vi "shutters activate.vi"() -> ()   [LabVIEW 2011]
doc: "Allows manual operation of laser and camera shutters on h-nu microscope"
uses:
  h-nu-ixon/Laser type.ctt
  h-nu-ixon/Emission filters.ctl
  h-nu-ixon/Filter wheel settings globals.vi
  hardware status globals.vi
panel:
  in  "L0 off1 2":bool
  in  "L0 ON 5":bool
  in  "Emission filter wheel":T1
  out "Status":bool
  in  "C off":bool
  in  "C ON":bool
  out "error out":errorcluster
  in  "All Lasers Off":bool
  in  "L0 off 4":bool
  in  "L0 off 3":bool
  in  "L0 off1":bool
  in  "L0 off 0":bool
  in  "L0 ON 4":bool
  in  "L0 ON 3":bool
  in  "L0 ON 2":bool
  in  "Stop":bool
  in  "L0 ON":bool
  out "Lasers Shutters Status":cluster{"Laser":T2, "Status":bool}[](array[cluster])=[{"Laser"=enum."Blue 488 nm", "Status"=FALSE}, {"Laser"=enum."Green 532 nm", "Status"=FALSE}, {"Laser"=enum."Orange 594 nm", "Status"=FALSE}, {"Laser"=enum."Red 633 nm", "Status"=FALSE}, {"Laser"=enum."IR 780", "Status"=FALSE}]
  # "Open"
  # "Close"
  # "Camera"
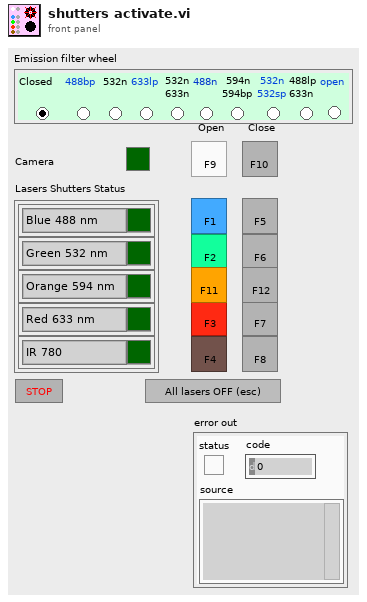
[diagram p1: front panel]
types:
  T1 = typedef "Emission filters.ctl" = enum32{" Closed ", "488bp ", "532n", "633lp ", "532n\n633n", "488n", "594n\n594bp", "532n\n532sp", "488lp\n633n", "open"}
  T2 = typedef "Laser type.ctt" = enum16{"Blue 488 nm", "Green 532 nm", "Orange 594 nm", "Red 633 nm", "IR 780"}
  T3 = enum16{"Blue 488 nm", "Green 532 nm", "Orange 594 nm", "Red 633 nm", "IR 780"}
  T4 = typedef "shutters status.ctl" = cluster{"Laser":T2, "Status":bool}[]
  T5 = enum16{"Blue 488 nm", "Green 532 nm", "Orange 594 nm", "Red 633 nm", "IR 780"}[]
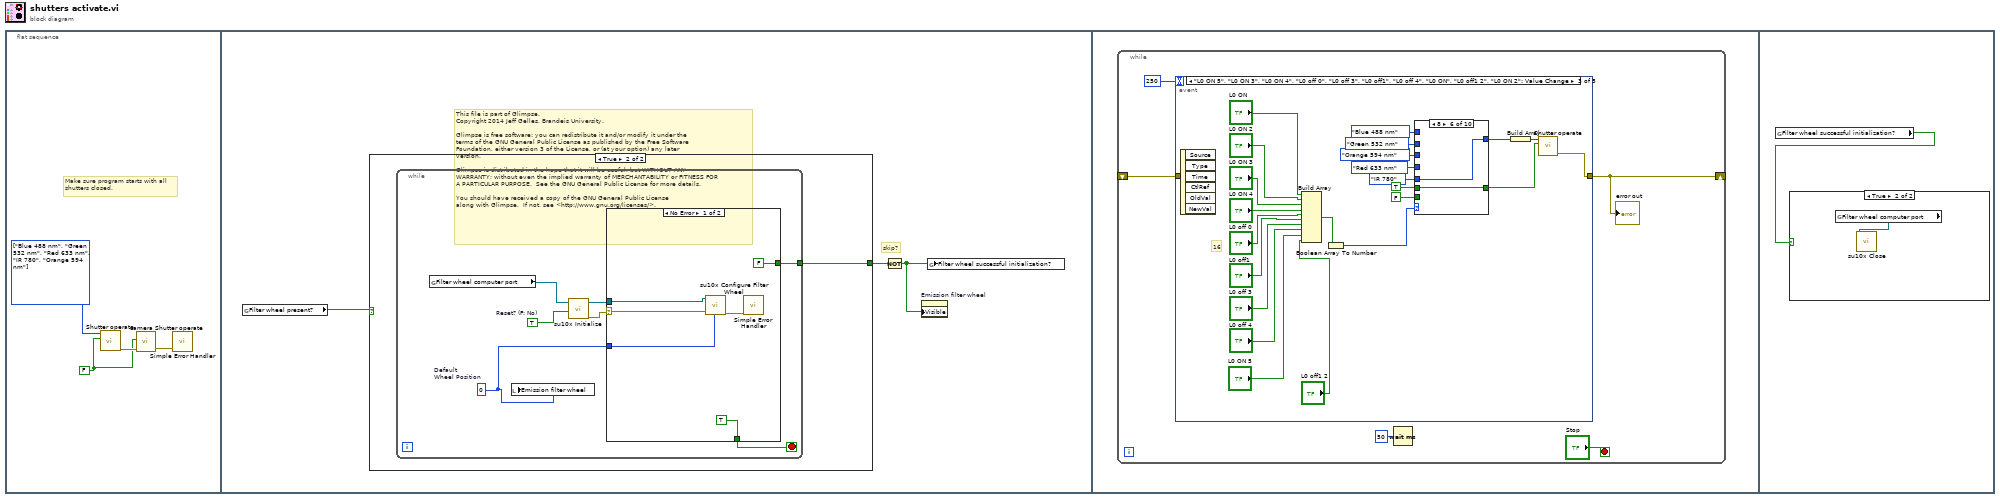
[diagram p0: block diagram]
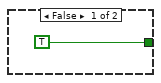
[diagram p2: hidden frame]
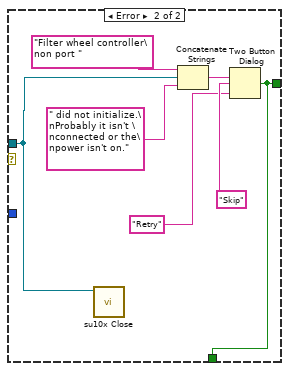
[diagram p3: hidden frame]
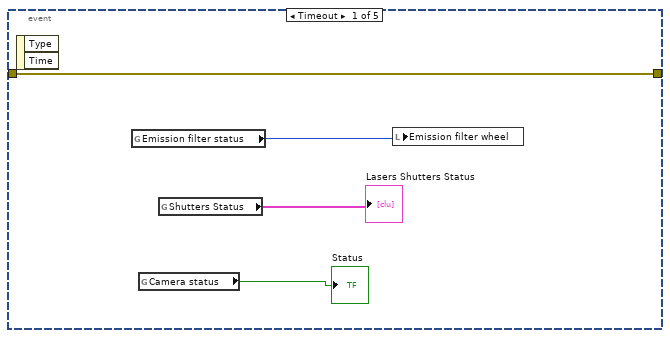
[diagram p4: hidden frame]
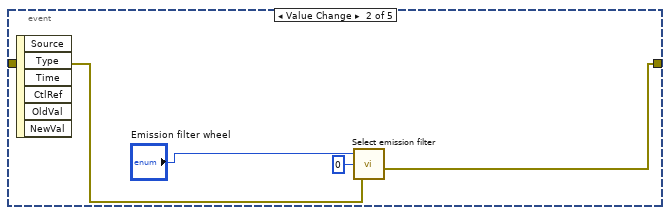
[diagram p5: hidden frame]
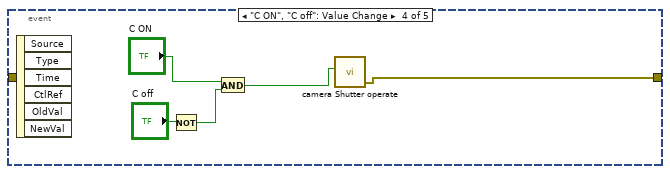
[diagram p15: hidden frame]
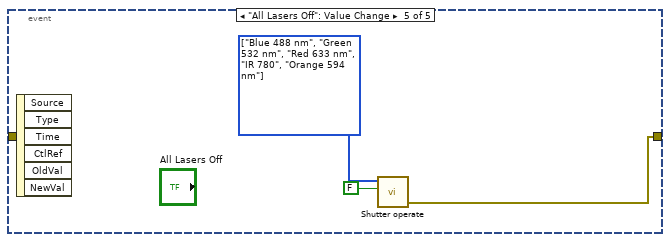
[diagram p16: hidden frame]
diagram:
  # "This file is part of Glimpse. \nCopyright 2014 Jeff Gelles, Brandeis University.    \n\nGlimpse is free software: you can redistribute it and/or modify it under the \nterms of the GNU General Public License as published by the Free Software \nFoundation, either version 3 of the License, or (at your option) any later \nversion.\n\nGlimpse is distributed in the hope that it will be useful, but WITHOUT ANY \nWARRANTY; without even the implied warranty of MERCHANTABILITY or FITNESS FOR \nA PARTICULAR PURPOSE.  See the GNU General Public License for more details.\n\nYou should have received a copy of the GNU General Public License\nalong with Glimpse.  If not, see <http://www.gnu.org/licenses/>."
  n1 = flat-sequence {
    frame #0 {
      w4 = T2[] [enum."Blue 488 nm", enum."Green 532 nm", enum."Red 633 nm", enum."IR 780", enum."Orange 594 nm"] items=["Blue 488 nm", "Green 532 nm", "Orange 594 nm", "Red 633 nm", "IR 780"] ("Shutters")
      w1 = FALSE
      # "Make sure program starts with all\nshutters closed."
      n2 = call "Shutter operate.vi"("Shutters"=w4, 2:w1) -> ("error out"=w3:errorcluster)  [unwired: 1 in, 5 out]
      n3 = call "camera Shutter operate.vi"("Open?"=w1, "error in"=w3) -> ("error out"=w2:errorcluster)  [unwired: 6 out]
      n4 = call <vilib>:"Simple Error Handler.vi"("error in (no error)"=w2) -> ()  [unwired: 4 in, 5 out]
    }
    frame #1 {
      # "skip?"
      n5 = global read "Filter wheel settings globals.vi" "Filter wheel present?"() -> (w5:bool)
      n6 = case shown="True" w5 {
        tunnel: [TRUE ("T button?") w9] -> w6
        frame False {
        }
        frame True {
          n7 = while {
            tunnel: [w11] -> w9
            stop <- w13 stop-if-true
            w10 = u8 0  # Default Wheel Position
            w15 = TRUE  # Reset? (F: No)
            n8 = global read "Filter wheel settings globals.vi" "Filter wheel computer port"() -> (w16:refnum<visa-resource-name>)
            n9 = local write "Emission filter wheel"(w10) -> ()
            n10 = call <instrlib>:"su10x Initialize.vi"("Reset? (F: No)"=w15, "VISA resource name"=w16) -> ("error out"=w14:errorcluster, "VISA resource name out"=w12:refnum<visa-resource-name>)  [unwired: 2 in, 6 out]
            n11 = case shown="No Error" w14 {
              selector: w14 -> [w21 _]
              tunnel: [TRUE w23] -> w13
              tunnel: w12 -> [w20 w24]
              tunnel: [FALSE ("T button?") w23] -> w11
              tunnel: w10 -> [w18 _]
              frame No Error {
                n12 = call <instrlib>:"su10x Configure Filter Wheel.vi"("Wheel Position (0)"=w18, "error in (no error)"=w21, "VISA resource name"=w20) -> ("error out"=w17:errorcluster)  [unwired: 2 in, 6 out]
                n13 = call <vilib>:"Simple Error Handler.vi"("error in (no error)"=w17) -> ()  [unwired: 1 in, 8 out]
              }
              frame Error {
                n14 = call <instrlib>:"su10x Close.vi"("VISA resource name"=w24) -> ()  [unwired: 1 in, 10 out]
                n15 = Concatenate Strings("Filter wheel controller\non port " ("string"), w24, " did not initialize.\nProbably it isn't \nconnected or the\npower isn't on." ("string")) -> (w29:string)
                n16 = Two Button Dialog(message=w29, 1:"Retry" ("F button name (\"Cancel\")"), 2:"Skip" ("T button name (\"OK\")")) -> (T button?=w23:bool)
              }
            }
          }
        }
      }
      n17 = Not(x=w6) -> (.not. x?=w7:bool)
      n18 = property on="Emission filter wheel" class="RadioBtnsControl (strict)"("Visible"=w7) -> ()  [unwired: 2 in, 2 out]
      n19 = global write "Filter wheel settings globals.vi" "Filter wheel successful initialization?"(w7) -> ()
    }
    frame #2 {
      n20 = while {
        shift-right: [w30] -> _
        shift-left: _ -> [w31]
        stop <- "Stop" stop-if-true
        n21 = event shown="[2] \"L0 ON 5\", \"L0 ON 3\", \"L0 ON 4\", \"L0 off 0\", \"L0 off 3\", \"L0 off1\", \"L0 off 4\", \"L0 ON\", \"L0 off1 2\", \"L0 ON 2\": Value Change" {
          selector: _ -> [_ _ _ _ _]
          dyn-events: _ -> [_ _ _ _ _]
          timeout: 250 -> [_ _ _ _ _]
          tunnel: [w37 w42 w46 w86 w91] -> w30
          tunnel: w31 -> [w37 w41 _ _ _]
          event Timeout {
            n22 = event-data() -> ()  [unwired: 3 out]
            n23 = global read "hardware status globals.vi" "Emission filter status"() -> (w35:T1)
            n24 = global read "hardware status globals.vi" "Camera status"() -> (→"Status":bool)
            n25 = global read "hardware status globals.vi" "Shutters Status"() -> (→"Lasers Shutters Status":T4)
            n26 = local write "Emission filter wheel"(w35) -> ()
          }
          event Value Change {
            n27 = event-data() -> ()  [unwired: 7 out]
            n28 = call "Select emission filter.vi"("Emission filter"="Emission filter wheel", "Time to wait\nafter filter change\n(ms)"=u32 0 ("Time to wait\nafter filter change\n(ms)"), "error in"=w41) -> ("error out"=w42:errorcluster)  [unwired: 3 out]
          }
          event "L0 ON 5", "L0 ON 3", "L0 ON 4", "L0 off 0", "L0 off 3", "L0 off1", "L0 off 4", "L0 ON", "L0 off1 2", "L0 ON 2": Value Change {
            # "16"
            n29 = event-data() -> ()  [unwired: 7 out]
            n30 = Build Array("L0 ON", "L0 ON 2", "L0 ON 3", "L0 ON 4", "L0 off 0", "L0 off1", "L0 off 3", "L0 off 4", "L0 ON 5", "L0 off1 2") -> (w57:bool[])
            n31 = Boolean Array To Number(Boolean array=w57) -> (number=w56:u32)
            n32 = case shown="8" w56 {
              tunnel: [w67 w68 w71 w73 w75 w77 w79 w81 w83 w85] -> w54
              tunnel: T3."Blue 488 nm" -> [w67 _ _ _ _ _ w79 _ _ _]
              tunnel: TRUE -> [w66 w69 _ w72 w74 w76 _ _ _ _]
              tunnel: [w66 w69 w70 w72 w74 w76 w78 w80 w82 w84] -> w51
              tunnel: T3."Green 532 nm" -> [_ _ _ w73 _ _ _ w81 _ _]
              tunnel: T3."Red 633 nm" -> [_ _ _ _ w75 _ _ _ w83 _]
              tunnel: T3."IR 780" -> [_ _ _ _ _ w77 _ _ _ w85]
              tunnel: FALSE -> [_ _ w70 _ _ _ w78 w80 w82 w84]
              tunnel: T3."Orange 594 nm" -> [_ w68 w71 _ _ _ _ _ _ _]
              frame 1, Default {
              }
              frame 256 {
              }
              frame 512 {
              }
              frame 2 {
              }
              frame 4 {
              }
              frame 8 {
              }
              frame 16 {
              }
              frame 32 {
              }
              frame 64 {
              }
              frame 128 {
              }
            }
            n33 = Build Array(w54) -> (w55:T5)
            n34 = call "Shutter operate.vi"("Shutters"=w55, 2:w51) -> ("error out"=w46:errorcluster)  [unwired: 1 in, 5 out]
          }
          event "C ON", "C off": Value Change {
            n35 = event-data() -> ()  [unwired: 7 out]
            n36 = Not(x="C off") -> (.not. x?=w89:bool)
            n37 = And(x="C ON", y=w89) -> (x .and. y?=w87:bool)
            n38 = call "camera Shutter operate.vi"("Open?"=w87) -> ("error out"=w86:errorcluster)  [unwired: 1 in, 6 out]
          }
          event "All Lasers Off": Value Change {
            w92 = T2[] [enum."Blue 488 nm", enum."Green 532 nm", enum."Red 633 nm", enum."IR 780", enum."Orange 594 nm"] items=["Blue 488 nm", "Green 532 nm", "Orange 594 nm", "Red 633 nm", "IR 780"] ("Shutters")
            n39 = event-data() -> ()  [unwired: 7 out]
            n40 = call "Shutter operate.vi"("Shutters"=w92, 2:FALSE) -> ("error out"=w91:errorcluster)  [unwired: 1 in, 5 out]
          }
        }
        "error out" <- w30
        n41 = Wait (ms)(milliseconds to wait=u32 50) -> ()  [unwired: 1 out]
      }
    }
    frame #3 {
      n42 = global read "Filter wheel settings globals.vi" "Filter wheel successful initialization?"() -> (w94:bool)
      n43 = case shown="True" w94 {
        frame False {
        }
        frame True {
          n44 = global read "Filter wheel settings globals.vi" "Filter wheel computer port"() -> (w95:refnum<visa-resource-name>)
          n45 = call <instrlib>:"su10x Close.vi"("VISA resource name"=w95) -> ()  [unwired: 1 in, 10 out]
        }
      }
    }
  }
